vi "Hlavny program FINAL.vi"() -> ()   [LabVIEW 2018]
uses:
  <vilib>/Utility/file.llb/Write Delimited Spreadsheet (DBL).vi
panel:
  out "Pomer":dbl
  out "ERR Inicial":bool
  out "ERR VISA FUN GEN":bool
  out "ERR VISA DAQ":bool
  out "Err konveryia na string":bool
  out "size(s)":i32
  out "(HB)max":dbl
  out "Retentivita":dbl
  out "Koercitivne pole":dbl
  out "Magneticka indukcia":dbl[](array[numeric])
  out "indukovane napatie":dbl[](array[numeric])
  out "Intezita mag pola":dbl[](array[numeric])
  out "Budiac prud":dbl[](array[numeric])
  in  "File IO":bool
  out "String fun gen idn?":string
  in  "FUN GEN IDN?":bool
  in  "VISA FUN GEN":refnum<visa-resource-name>
  out "Pocet bodov":dbl
  out "Data user defined":string
  in  "Vlastny priebeh":bool
  in  "Typ priebehu":string(combo)="0"
  in  "Frekvencia":i16(knob)=500 scale=0.0..600.0
  in  "Magnetovací prúd":dbl(knob)=0.5 scale=0.0..1.5 scale format="%#_2f"
  out "Pocet ERR":dbl
  out "Intenzita mag. pola":waveform(dbl)(graph)
  out "ERR 2":bool
  out "DATA":string
  out "ERR 1":bool
  in  "N2":dbl=20.0
  in  "N1":dbl=131.0
  in  "h":dbl=0.005
  in  "r2":dbl=0.0125
  in  "r1":dbl=0.01
  in  "Rn":dbl=4.7
  in  "Demangnetizacia":bool
  out "Slucka":cluster{dbl, dbl}[](graph)
  out "String":string
  in  "daq IDN?":bool
  out "Indukuvane napatie":waveform(dbl)(graph)
  out "Magneticka indukcia":waveform(dbl)(graph)
  out "Budiaci prud":waveform(dbl)(graph)
  in  "DAQ":refnum<visa-resource-name>
  in  "Meranie":bool
  in  "stop":bool
  # "Prametre vzorky"
  # "Uh*N1"
  # "2*Pi"
  # "2*pi*rs"
  # "2*pi*rs*Rn"
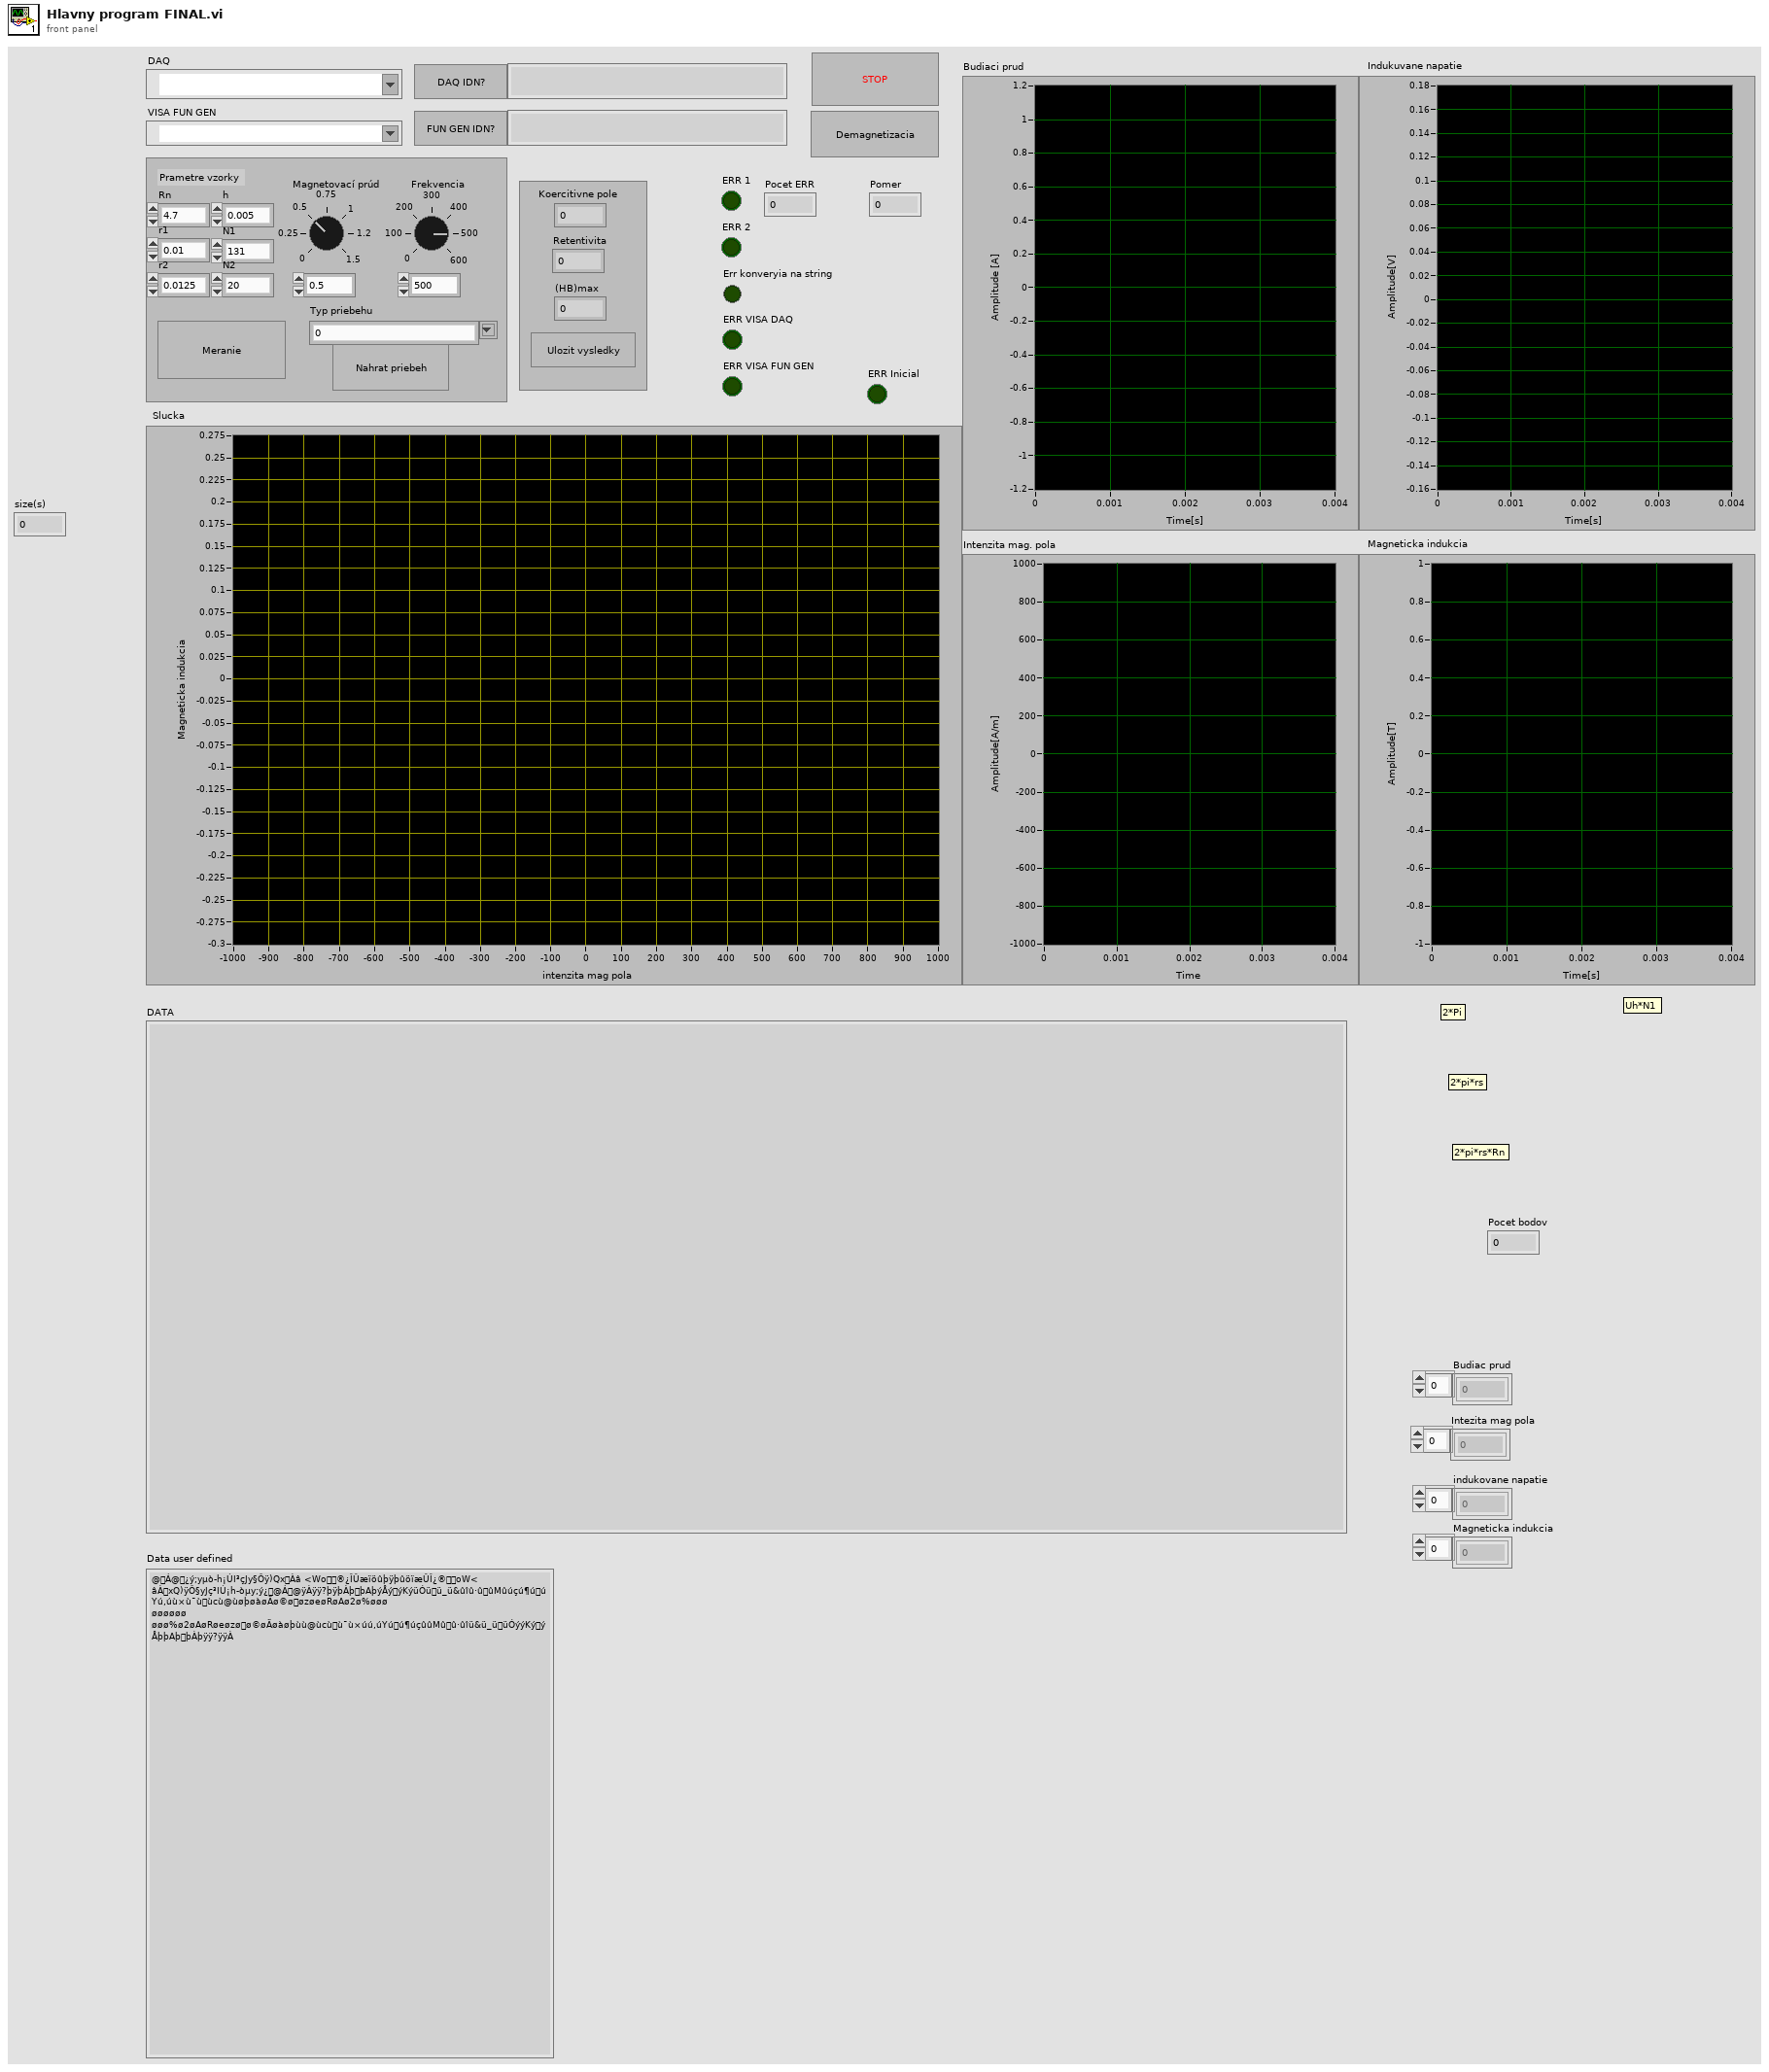
[diagram p1: front panel]
types:
  T1 = enum16{"big-endian, network order", "native, host order", "little-endian"}
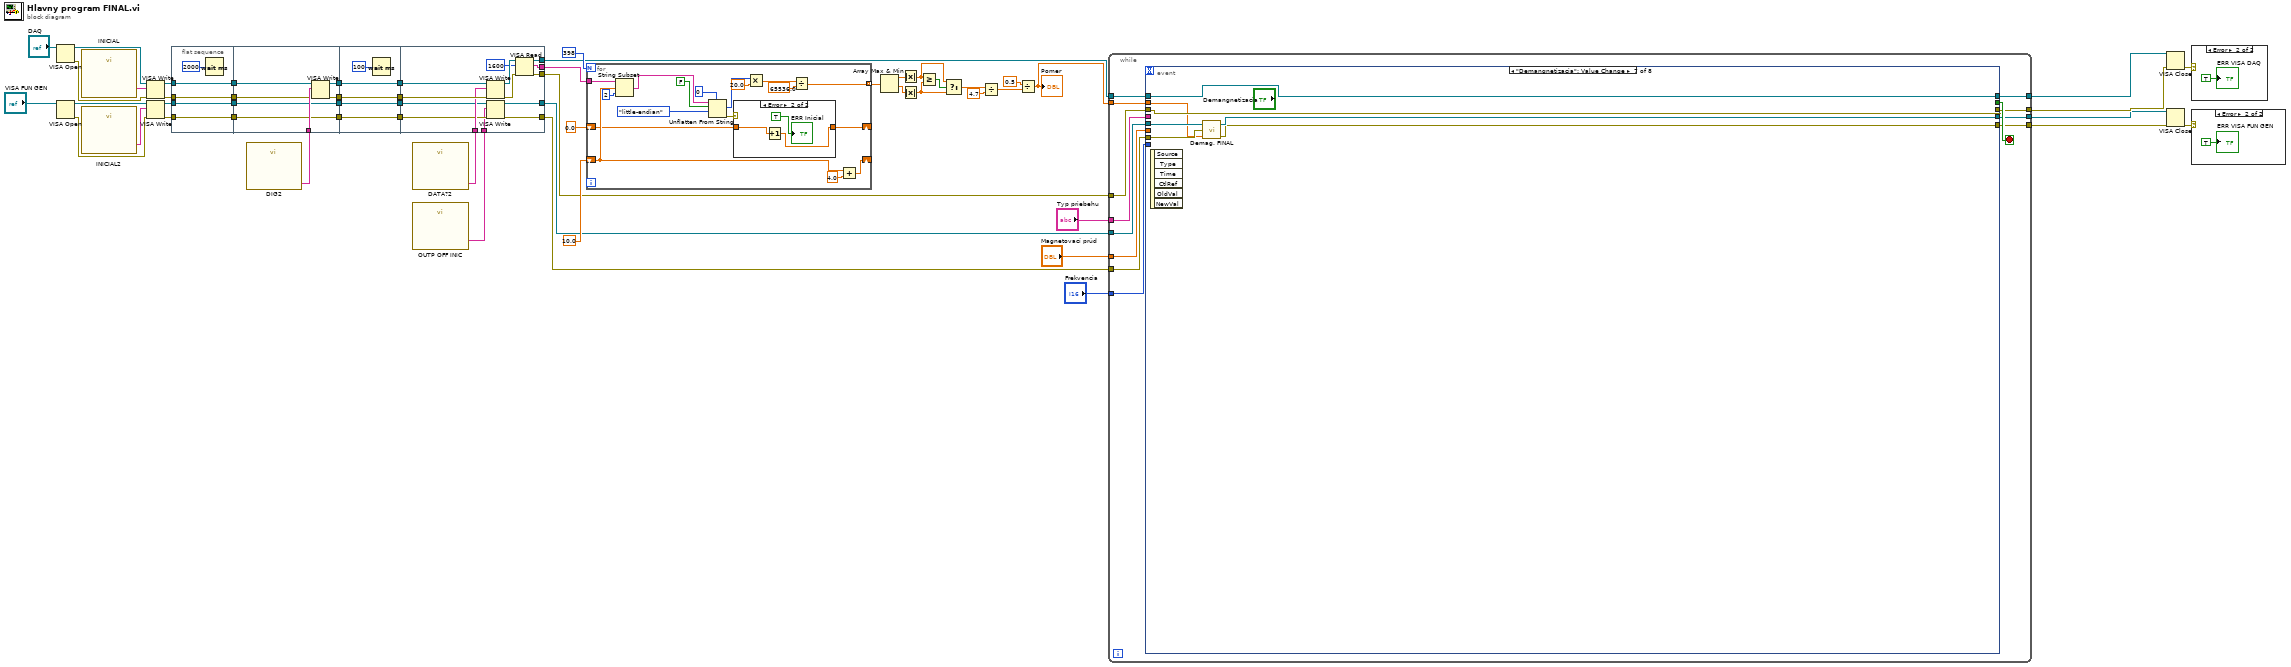
[diagram p0: block diagram]
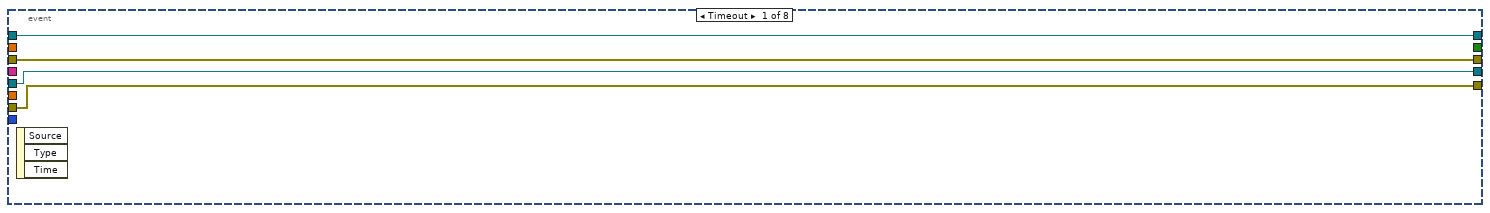
[diagram p5: hidden frame]
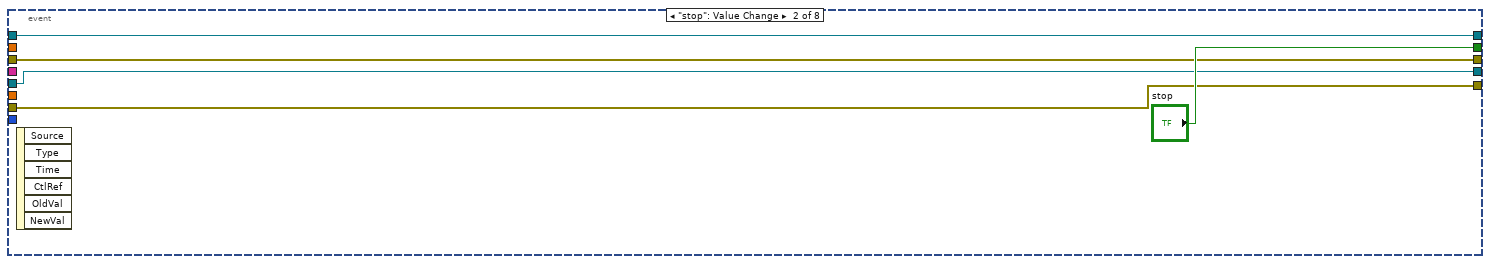
[diagram p6: hidden frame]
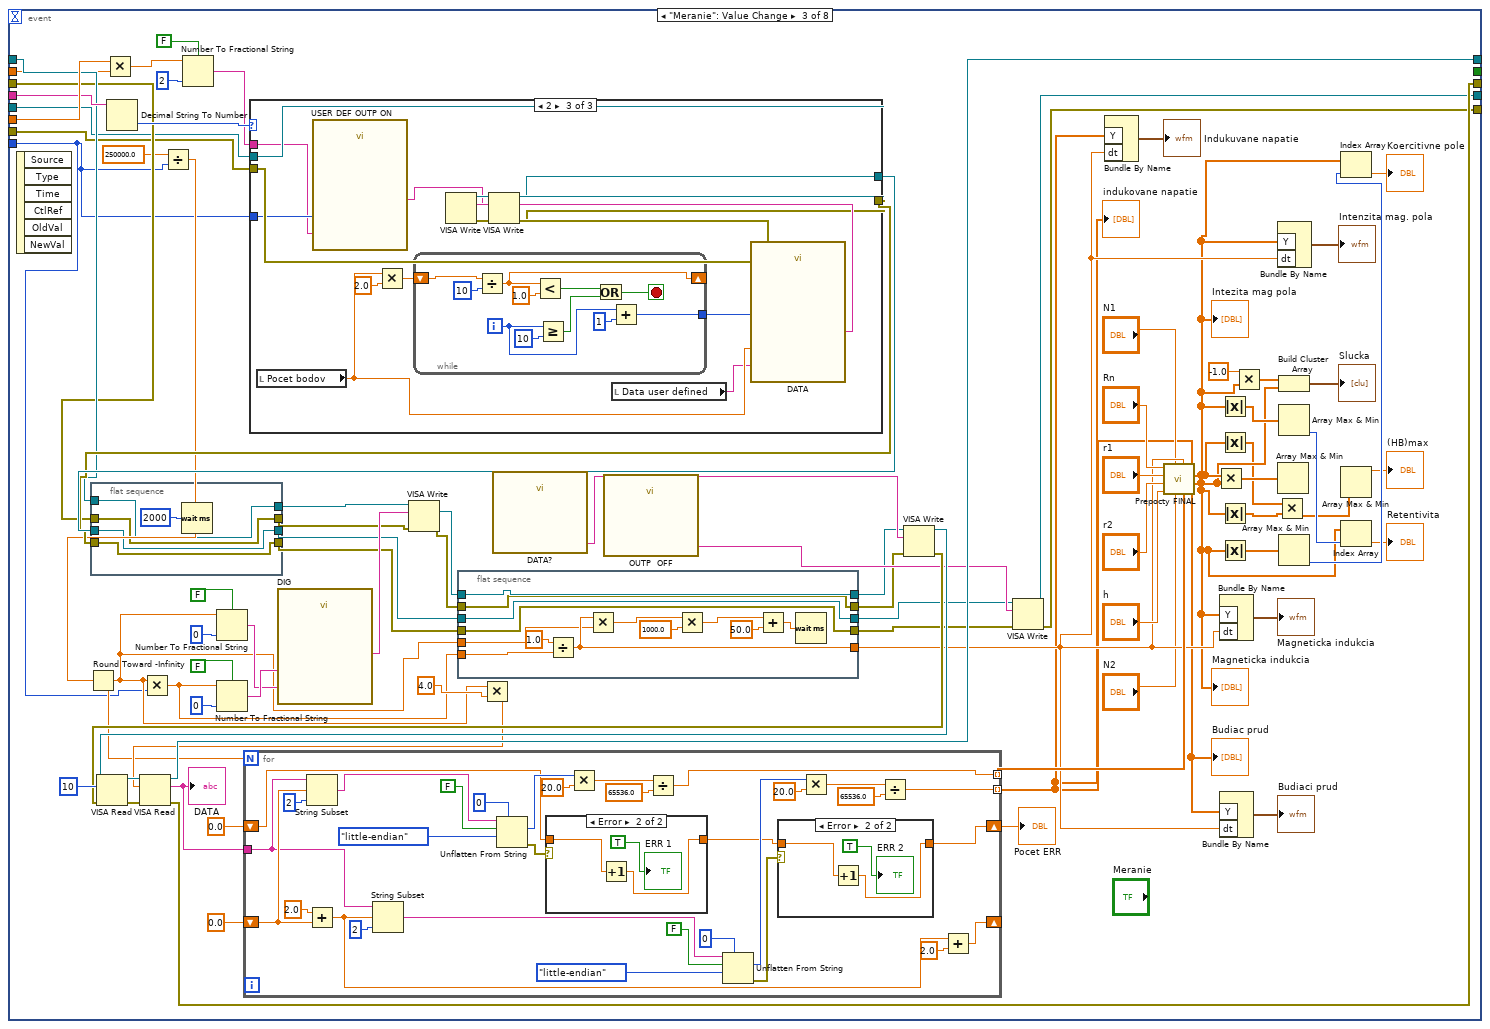
[diagram p7: hidden frame]
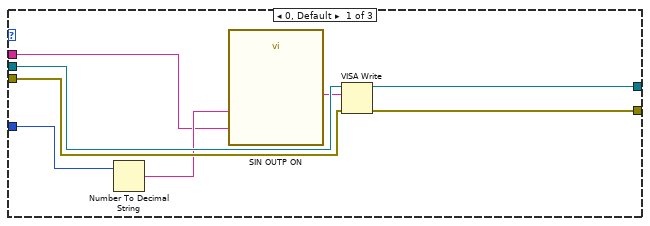
[diagram p8: hidden frame]
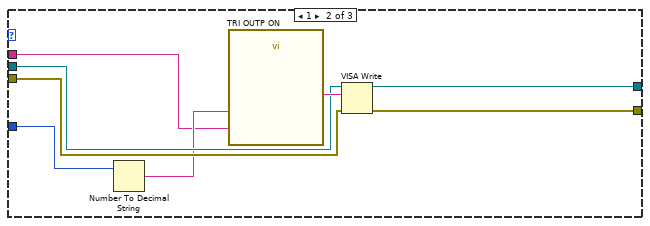
[diagram p9: hidden frame]
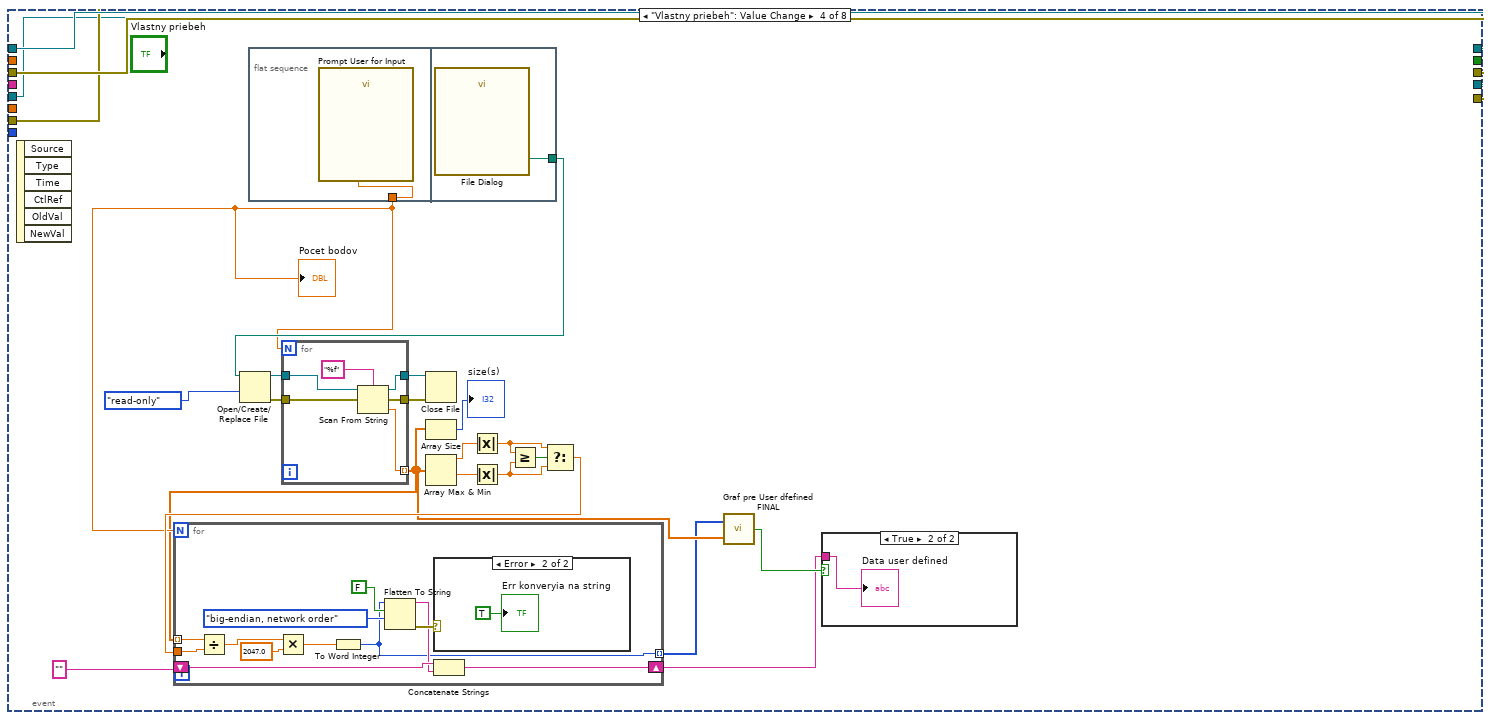
[diagram p12: hidden frame]
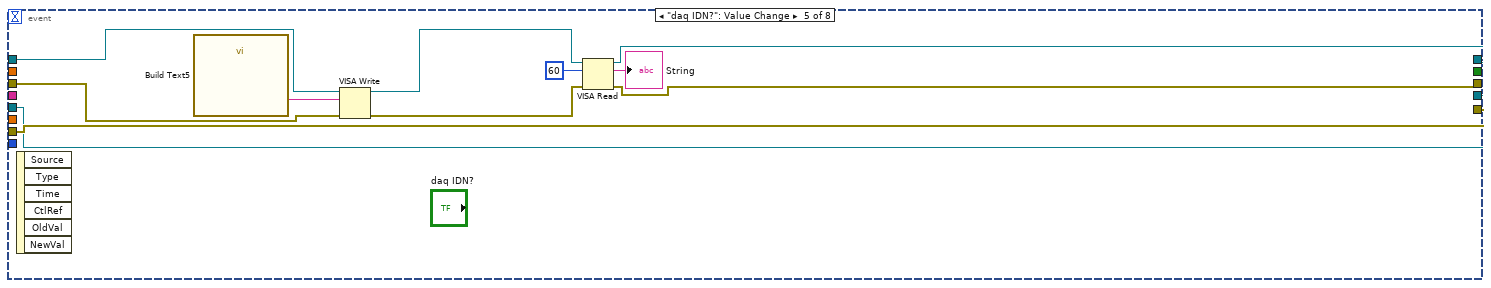
[diagram p15: hidden frame]
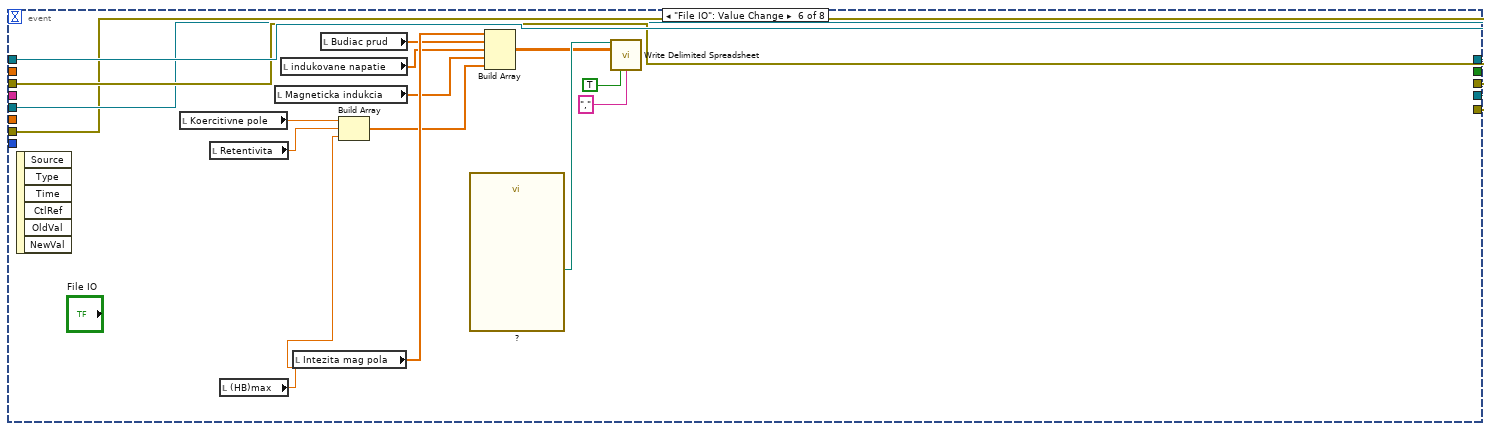
[diagram p16: hidden frame]
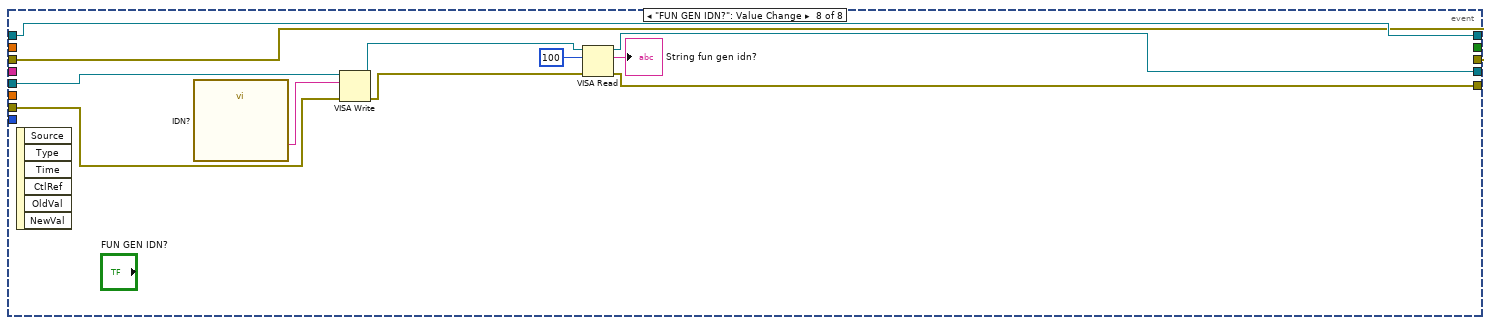
[diagram p17: hidden frame]
diagram:
  n1 = VISA Open(VISA resource name="DAQ") -> (VISA resource name=w52:refnum<visa-resource-name>, error out=w51:errorcluster)  [unwired: 4 in]
  n2 = VISA Open(VISA resource name="VISA FUN GEN") -> (VISA resource name=w43:refnum<visa-resource-name>, error out=w42:errorcluster)  [unwired: 4 in]
  n3 = call "INICIAL"() -> ("Result"=w50:string)  [unwired: 14 in, 1 out]
  n4 = call "INICIAL2"() -> ("Result"=w41:string)  [unwired: 14 in, 1 out]
  n5 = VISA Write(VISA resource name=w52, write buffer=w50, error in (no error)=w51) -> (VISA resource name out=w12:refnum<visa-resource-name>, error out=w13:errorcluster)  [unwired: 1 out]
  n6 = VISA Write(VISA resource name=w43, write buffer=w41, error in (no error)=w42) -> (VISA resource name out=w11:refnum<visa-resource-name>, error out=w10:errorcluster)  [unwired: 1 out]
  n7 = flat-sequence {
    tunnel: [w59] -> w38
    tunnel: w13 -> [w59]
    tunnel: [w58] -> w37
    tunnel: w12 -> [w58]
    tunnel: [w57] -> w36
    tunnel: w11 -> [w57]
    tunnel: [w56] -> w35
    tunnel: w10 -> [w56]
    tunnel: w26 -> [w67]
    tunnel: w38 -> [w66]
    tunnel: w37 -> [w64]
    tunnel: [w65] -> w34
    tunnel: [w63] -> w33
    tunnel: [w62] -> w32
    tunnel: w36 -> [w62]
    tunnel: [w61] -> w31
    tunnel: w35 -> [w61]
    tunnel: w34 -> [w72]
    tunnel: w33 -> [w71]
    tunnel: [w72] -> w30
    tunnel: [w71] -> w29
    tunnel: [w69] -> w28
    tunnel: w32 -> [w69]
    tunnel: [w68] -> w27
    tunnel: w31 -> [w68]
    tunnel: w30 -> [w85]
    tunnel: w29 -> [w86]
    tunnel: w25 -> [w84]
    tunnel: [w80] -> w24
    tunnel: [w79] -> w5
    tunnel: [w78] -> w6
    tunnel: w28 -> [w77]
    tunnel: w27 -> [w76]
    tunnel: [w75] -> w3
    tunnel: [w74] -> w4
    tunnel: w21 -> [w73]
    frame #0 {
      n8 = Wait (ms)(milliseconds to wait=u32 2000) -> ()  [unwired: 1 out]
    }
    frame #1 {
      n9 = VISA Write(VISA resource name=w64, write buffer=w67, error in (no error)=w66) -> (VISA resource name out=w63:refnum<visa-resource-name>, error out=w65:errorcluster)  [unwired: 1 out]
    }
    frame #2 {
      n10 = Wait (ms)(milliseconds to wait=u32 100) -> ()  [unwired: 1 out]
    }
    frame #3 {
      n11 = VISA Write(VISA resource name=w86, write buffer=w84, error in (no error)=w85) -> (VISA resource name out=w83:refnum<visa-resource-name>, error out=w82:errorcluster)  [unwired: 1 out]
      n12 = VISA Write(VISA resource name=w77, write buffer=w73, error in (no error)=w76) -> (VISA resource name out=w75:refnum<visa-resource-name>, error out=w74:errorcluster)  [unwired: 1 out]
      n13 = VISA Read(VISA resource name=w83, byte count=u32 1600, error in (no error)=w82) -> (VISA resource name out=w79:refnum<visa-resource-name>, read buffer=w80:string, error out=w78:errorcluster)  [unwired: 1 out]
    }
  }
  n14 = call "DIG2"() -> ("Result"=w26:string)  [unwired: 14 in, 1 out]
  n15 = call "DATA?2"() -> ("Result"=w25:string)  [unwired: 14 in, 1 out]
  n16 = call "OUTP OFF INIC"() -> ("Result"=w21:string)  [unwired: 14 in, 1 out]
  n17 = for {
    N: 398 -> [_]
    shift-right: [w102] -> _
    shift-left: 10.0 -> [w88]
    shift-right: [w92] -> _
    shift-left: 0.0 -> [w87]
    tunnel: w24 -> [w89]
    tunnel: [w90] -> w2 mode=indexing
    n18 = String Subset(string=w89, offset (0)=w88, length (rest)=2 ("length (rest)")) -> (substring=w93:string)
    n19 = Unflatten From String(type=i16 0, binary string=w93, data includes array or string size? (T)=FALSE, byte order (0:big-endian, network order)=T1."little-endian") -> (value=w96:i16, error out=w91:errorcluster)  [unwired: 1 in, 1 out]
    n20 = case shown="Error" w91 {
      tunnel: [w104 w106] -> w92
      tunnel: w87 -> [w104 w105]
      frame No Error {
      }
      frame Error {
        n21 = Increment(x=w105) -> (x+1=w106:dbl)
        "ERR Inicial" <- TRUE ("ERR")
      }
    }
    n22 = Multiply(x=w96, y=20.0) -> (x*y=w100:dbl)
    n23 = Divide(x=w100, y=65536.0) -> (x/y=w90:dbl)
    n24 = Add(x=w88, y=4.0) -> (x+y=w102:dbl)
  }
  n25 = Array Max & Min(array=w2) -> (max value=w20:dbl, min value=w19:dbl)  [unwired: 2 out]
  n26 = Absolute Value(x=w20) -> (abs(x)=w18:dbl)
  n27 = Absolute Value(x=w19) -> (abs(x)=w17:dbl)
  n28 = Greater Or Equal?(x=w18, y=w17) -> (x >= y?=w16:bool)
  n29 = Select(t=w18, s=w16, f=w17) -> (s? t:f=w9:dbl)
  n30 = Divide(x=w9, y=4.7) -> (x/y=w7:dbl)
  n31 = Divide(x=0.5, y=w7) -> (x/y=w1:dbl)
  "Pomer" <- w1
  n32 = while {
    tunnel: w5 -> [w119]
    tunnel: w6 -> [w118]
    tunnel: [w117] -> w54
    tunnel: [w116] -> w53
    tunnel: "Magnetovací prúd" -> [w115]
    tunnel: "Frekvencia" -> [w113]
    tunnel: "Typ priebehu" -> [w114]
    tunnel: w3 -> [w112]
    tunnel: w4 -> [w111]
    tunnel: [w110] -> w45
    tunnel: [w109] -> w44
    tunnel: w1 -> [w108]
    stop <- w120 stop-if-true
    n33 = event shown="[6] \"Demangnetizacia\": Value Change" {
      selector: _ -> [_ _ _ _ _ _ _ _]
      dyn-events: _ -> [_ _ _ _ _ _ _ _]
      timeout: _ -> [_ _ _ _ _ _ _ _]
      tunnel: [_ "stop" _ _ _ _ _ _] -> w120
      tunnel: w119 -> [w124 w128 w170 w333 w367 w383 w390 w401]
      tunnel: w118 -> [w121 w125 w168 w334 w366 w382 w389 w397]
      tunnel: [w124 w128 w198 w333 w360 w383 w390 w401] -> w117
      tunnel: [w121 w125 w197 w334 w359 w382 w389 w397] -> w116
      tunnel: w115 -> [_ _ w187 _ _ _ _ _]
      tunnel: w114 -> [_ _ w186 _ _ _ _ _]
      tunnel: w113 -> [_ _ w131 _ _ _ _ _]
      tunnel: w112 -> [w122 w126 w165 w330 w357 w381 w388 w399]
      tunnel: w111 -> [w123 w127 w164 w331 w358 w380 w387 w398]
      tunnel: [w122 w126 w158 w330 w357 w381 w386 w394] -> w110
      tunnel: [w123 w127 w159 w331 w358 w380 w385 w393] -> w109
      tunnel: w108 -> [_ _ w130 _ _ _ w384 _]
      event Timeout {
        n34 = event-data() -> ()  [unwired: 1 in, 3 out]
      }
      event "stop": Value Change {
        n35 = event-data() -> ()  [unwired: 1 in, 6 out]
      }
      event "Meranie": Value Change {
        n36 = event-data() -> ()  [unwired: 1 in, 6 out]
        n37 = flat-sequence {
          tunnel: [w311] -> w161
          tunnel: w183 -> [w311]
          tunnel: [w310] -> w162
          tunnel: w182 -> [w310]
          tunnel: [w308] -> w171
          tunnel: w170 -> [w308]
          tunnel: [w307] -> w169
          tunnel: w168 -> [w307]
          frame #0 {
            n38 = Wait (ms)(milliseconds to wait=u32 2000) -> ()  [unwired: 1 out]
          }
        }
        n39 = Multiply(x=w187, y=w130) -> (x*y=w188:dbl)
        n40 = Decimal String To Number(string=w186) -> (number=w185:i32)  [unwired: 2 in, 1 out]
        n41 = Divide(x=250000.0, y=w131) -> (x/y=w142:dbl)
        n42 = Round Toward -Infinity(1:w142) -> (0:w133:dbl)
        n43 = Multiply(x=w133, y=w131) -> (x*y=w132:dbl)
        n44 = Number To Fractional String(use system decimal point (T)=FALSE, number=w188, precision (6)=i16 2) -> (F-format string=w184:string)  [unwired: 1 in]
        n45 = Number To Fractional String(use system decimal point (T)=FALSE, number=w133, precision (6)=i16 0) -> (F-format string=w137:string)  [unwired: 1 in]
        n46 = Number To Fractional String(use system decimal point (T)=FALSE, number=w132, precision (6)=i16 0) -> (F-format string=w138:string)  [unwired: 1 in]
        n47 = case shown="2" w185 {
          tunnel: w184 -> [w213 w221 w229]
          tunnel: w164 -> [w219 w226 w242]
          tunnel: w165 -> [w218 w225 w243]
          tunnel: [w216 w223 w238] -> w183
          tunnel: [w217 w224 w237] -> w182
          tunnel: w131 -> [w220 w228 w230]
          frame 0, Default {
            n48 = Number To Decimal String(number=w220) -> (decimal integer string=w214:string)  [unwired: 1 in]
            n49 = call "SIN OUTP ON"("Frekv"=w214, "ampl"=w213) -> ("Result"=w215:string)  [unwired: 12 in, 1 out]
            n50 = VISA Write(VISA resource name=w218, write buffer=w215, error in (no error)=w219) -> (VISA resource name out=w216:refnum<visa-resource-name>, error out=w217:errorcluster)  [unwired: 1 out]
          }
          frame 1 {
            n51 = Number To Decimal String(number=w228) -> (decimal integer string=w222:string)  [unwired: 1 in]
            n52 = call "TRI OUTP ON"("Frekv"=w222, "ampl"=w221) -> ("Result"=w227:string)  [unwired: 12 in, 1 out]
            n53 = VISA Write(VISA resource name=w225, write buffer=w227, error in (no error)=w226) -> (VISA resource name out=w223:refnum<visa-resource-name>, error out=w224:errorcluster)  [unwired: 1 out]
          }
          frame 2 {
            n54 = local read "Pocet bodov"() -> (w233:dbl)
            n55 = call "USER DEF OUTP ON"("frekv"=w230, "ampl"=w229) -> ("Result"=w236:string)  [unwired: 12 in, 1 out]
            n56 = Multiply(x=w233, y=2.0) -> (x*y=w234:dbl)
            n57 = while {
              shift-right: [w247] -> _
              shift-left: w234 -> [w249]
              tunnel: [w244] -> w231
              i -> [w246]
              stop <- w250 stop-if-true
              n58 = Divide(x=w249, y=10) -> (x/y=w247:dbl)
              n59 = Less?(x=w247, y=1.0) -> (x < y?=w253:bool)
              n60 = Greater Or Equal?(x=w246, y=10) -> (x >= y?=w252:bool)
              n61 = Or(x=w253, y=w252) -> (x .or. y?=w250:bool)
              n62 = Add(x=w246, y=1) -> (x+y=w244:i32)
            }
            n63 = local read "Data user defined"() -> (w232:string)
            n64 = call "DATA"("pocetdig"=w231, "pocetbod"=w233, "data"=w232) -> ("Result"=w241:string)  [unwired: 11 in, 1 out]
            n65 = VISA Write(VISA resource name=w243, write buffer=w241, error in (no error)=w242) -> (VISA resource name out=w240:refnum<visa-resource-name>, error out=w239:errorcluster)  [unwired: 1 out]
            n66 = VISA Write(VISA resource name=w240, write buffer=w236, error in (no error)=w239) -> (VISA resource name out=w238:refnum<visa-resource-name>, error out=w237:errorcluster)  [unwired: 1 out]
          }
        }
        n67 = call "DIG"("frekv"=w138, "body"=w137) -> ("Result"=w212:string)  [unwired: 12 in, 1 out]
        n68 = VISA Write(VISA resource name=w171, write buffer=w212, error in (no error)=w169) -> (VISA resource name out=w211:refnum<visa-resource-name>, error out=w210:errorcluster)  [unwired: 1 out]
        n69 = flat-sequence {
          tunnel: w211 -> [w303]
          tunnel: [w303] -> w167
          tunnel: w210 -> [w302]
          tunnel: [w302] -> w166
          tunnel: [w301] -> w176
          tunnel: [w297] -> w163
          tunnel: w162 -> [w297]
          tunnel: [w296] -> w160
          tunnel: w161 -> [w296]
          tunnel: w132 -> [w295]
          tunnel: w133 -> [w294]
          frame #0 {
            n70 = Divide(x=1.0, y=w295) -> (x/y=w301:dbl)
            n71 = Multiply(x=w301, y=w294) -> (x*y=w300:dbl)
            n72 = Multiply(x=w300, y=1000.0) -> (x*y=w298:dbl)
            n73 = Add(x=w298, y=50.0) -> (x+y=w304:dbl)
            n74 = Wait (ms)(milliseconds to wait=w304) -> ()  [unwired: 1 out]
          }
        }
        n75 = Multiply(x=w133, y=4.0) -> (x*y=w134:dbl)
        n76 = call "DATA?"() -> ("Result"=w196:string)  [unwired: 14 in, 1 out]
        n77 = call "OUTP  OFF"() -> ("Result"=w195:string)  [unwired: 14 in, 1 out]
        n78 = VISA Write(VISA resource name=w167, write buffer=w196, error in (no error)=w166) -> (VISA resource name out=w204:refnum<visa-resource-name>, error out=w203:errorcluster)  [unwired: 1 out]
        n79 = VISA Read(VISA resource name=w204, byte count=u32 10, error in (no error)=w203) -> (VISA resource name out=w202:refnum<visa-resource-name>, error out=w201:errorcluster)  [unwired: 2 out]
        n80 = VISA Read(VISA resource name=w202, byte count=w134, error in (no error)=w201) -> (VISA resource name out=w198:refnum<visa-resource-name>, read buffer=w194:string, error out=w197:errorcluster)  [unwired: 1 out]
        "DATA" <- w194
        n81 = for {
          N: w133 -> [_]
          shift-right: [w277] -> _
          shift-left: 0.0 -> [w267]
          shift-right: [w261] -> w191
          shift-left: 0.0 -> [w275]
          tunnel: w194 -> [w256]
          tunnel: [w259] -> w157 mode=indexing
          tunnel: [w258] -> w177 mode=indexing
          n82 = String Subset(string=w256, offset (0)=w267, length (rest)=2 ("length (rest)")) -> (substring=w276:string)
          n83 = Add(x=2.0, y=w267) -> (x+y=w257:dbl)
          n84 = String Subset(string=w256, offset (0)=w257, length (rest)=2 ("length (rest)")) -> (substring=w264:string)
          n85 = Unflatten From String(type=i16 0, binary string=w276, data includes array or string size? (T)=FALSE, byte order (0:big-endian, network order)=T1."little-endian") -> (value=w280:i16, error out=w263:errorcluster)  [unwired: 1 in, 1 out]
          n86 = case shown="Error" w263 {
            tunnel: [w290 w292] -> w262
            tunnel: w275 -> [w290 w291]
            frame No Error {
            }
            frame Error {
              n87 = Increment(x=w291) -> (x+1=w292:dbl)
              "ERR 1" <- TRUE ("ERR")
            }
          }
          n88 = Multiply(x=w280, y=20.0) -> (x*y=w284:dbl)
          n89 = Divide(x=w284, y=65536.0) -> (x/y=w258:dbl)
          n90 = Unflatten From String(type=i16 0, binary string=w264, data includes array or string size? (T)=FALSE, byte order (0:big-endian, network order)=T1."little-endian") -> (value=w269:i16, error out=w260:errorcluster)  [unwired: 1 in, 1 out]
          n91 = case shown="Error" w260 {
            tunnel: [w286 w288] -> w261
            tunnel: w262 -> [w286 w287]
            frame No Error {
            }
            frame Error {
              n92 = Increment(x=w287) -> (x+1=w288:dbl)
              "ERR 2" <- TRUE ("ERR")
            }
          }
          n93 = Multiply(x=w269, y=20.0) -> (x*y=w273:dbl)
          n94 = Divide(x=w273, y=65536.0) -> (x/y=w259:dbl)
          n95 = Add(x=w257, y=2.0) -> (x+y=w277:dbl)
        }
        "Pocet ERR" <- w191
        "indukovane napatie" <- w157
        n96 = VISA Write(VISA resource name=w160, write buffer=w195, error in (no error)=w163) -> (VISA resource name out=w158:refnum<visa-resource-name>, error out=w159:errorcluster)  [unwired: 1 out]
        n97 = Bundle By Name("Y"=w157, "dt"=w176) -> (→"Indukuvane napatie":waveform(dbl))  [unwired: 1 in]
        n98 = call "Prepocty FINAL.vi"("Ui"=w157, "Uh"=w177, "dt"=w176, "N2"="N2", "N1"="N1", "h"="h", "r2"="r2", "r1"="r1", "Rn"="Rn") -> ("I"=w173:dbl[], "B"=w148:dbl[], "H"=w149:dbl[])
        "Budiac prud" <- w173
        "Intezita mag pola" <- w149
        "Magneticka indukcia" <- w148
        n99 = Multiply(x=w149, y=w148) -> (x*y=w150:dbl[])
        n100 = Absolute Value(x=w149) -> (abs(x)=w154:dbl[])
        n101 = Absolute Value(x=w149) -> (abs(x)=w147:dbl[])
        n102 = Absolute Value(x=w148) -> (abs(x)=w146:dbl[])
        n103 = Absolute Value(x=w148) -> (abs(x)=w156:dbl[])
        n104 = Bundle By Name("Y"=w148, "dt"=w176) -> (→"Magneticka indukcia":waveform(dbl))  [unwired: 1 in]
        n105 = Bundle By Name("Y"=w173, "dt"=w176) -> (→"Budiaci prud":waveform(dbl))  [unwired: 1 in]
        n106 = Multiply(x=-1.0, y=w149) -> (x*y=w172:dbl[])
        n107 = Multiply(x=w147, y=w146) -> (x*y=w145:dbl[])
        n108 = Bundle By Name("Y"=w149, "dt"=w176) -> (→"Intenzita mag. pola":waveform(dbl))  [unwired: 1 in]
        n109 = Array Max & Min(array=w150) -> ()  [unwired: 4 out]
        n110 = Build Cluster Array(w172, w148) -> (→"Slucka":cluster{dbl, dbl}[])
        n111 = Array Max & Min(array=w154) -> (min index (indices)=w153:i32)  [unwired: 3 out]
        n112 = Array Max & Min(array=w156) -> (min index (indices)=w155:i32)  [unwired: 3 out]
        n113 = Index Array(array=w149, index=w155) -> (element=→"Koercitivne pole":dbl)
        n114 = Array Max & Min(array=w145) -> (max value=→"(HB)max":dbl)  [unwired: 3 out]
        n115 = Index Array(array=w148, index=w153) -> (element=→"Retentivita":dbl)
      }
      event "Vlastny priebeh": Value Change {
        n116 = event-data() -> ()  [unwired: 1 in, 6 out]
        n117 = Open/Create/Replace File(file path (use dialog)=w316, access (0:read/write)=enum16{"read/write", "read-only", "write-only"}."read-only") -> (refnum out=w328:refnum<file>, error out=w327:errorcluster)  [unwired: 4 in, 1 out]
        n118 = flat-sequence {
          tunnel: [w355] -> w315
          tunnel: [w356] -> w316
          frame #0 {
            n119 = call "Prompt User for Input"() -> ("Pocet bodov"=w355:dbl)  [unwired: 17 in, 2 out]
          }
          frame #1 {
            n120 = call "File Dialog"() -> ("selected path"=w356:path)  [unwired: 12 in, 3 out]
          }
        }
        n121 = for {
          N: w315 -> [_]
          tunnel: w328 -> [w350]
          tunnel: w327 -> [w349]
          tunnel: [w353] -> w325
          tunnel: [w352] -> w326
          tunnel: [w348] -> w314 mode=indexing
          n122 = Scan From String("%f" ("format string"), w350, w349) -> (w353:refnum<file>, w352:errorcluster, output 1=w348:dbl)  [unwired: 1 in]
        }
        n123 = Close File(refnum=w325, error in=w326) -> ()  [unwired: 2 out]
        n124 = Array Size(array=w314) -> (size(s)=→"size(s)":i32)
        n125 = Array Max & Min(array=w314) -> (max value=w323:dbl, min value=w322:dbl)  [unwired: 2 out]
        n126 = Absolute Value(x=w323) -> (abs(x)=w320:dbl)
        n127 = Absolute Value(x=w322) -> (abs(x)=w319:dbl)
        n128 = Greater Or Equal?(x=w320, y=w319) -> (x >= y?=w321:bool)
        n129 = Select(t=w320, s=w321, f=w319) -> (s? t:f=w318:dbl)
        n130 = for {
          N: w315 -> [_]
          tunnel: w318 -> [w342]
          tunnel: w314 -> [w343] mode=indexing
          shift-right: [w338] -> w312
          shift-left: "" -> [w337]
          tunnel: [w335] -> w313 mode=indexing
          n131 = Divide(x=w343, y=w342) -> (x/y=w341:dbl)
          n132 = Multiply(x=w341, y=2047.0) -> (x*y=w339:dbl)
          n133 = To Word Integer(number=w339) -> (16bit integer=w335:i16)
          n134 = Flatten To String(anything=w335, prepend array or string size? (T)=FALSE, byte order (0:big-endian, network order)=T1."big-endian, network order") -> (data string=w336:string, error out=w346:errorcluster)  [unwired: 1 in, 1 out]
          n135 = case shown="Error" w346 {
            frame No Error {
            }
            frame Error {
              "Err konveryia na string" <- TRUE ("Err konveryia na string")
            }
          }
          n136 = Concatenate Strings(w337, w336) -> (w338:string)
        }
        n137 = call "Graf pre User dfefined FINAL.vi"("Array"=w314, "Array 2"=w313) -> ("Boolean"=w332:bool)
        n138 = case shown="True" w332 {
          tunnel: w312 -> [_ w354]
          frame False {
          }
          frame True {
            "Data user defined" <- w354
          }
        }
        "Pocet bodov" <- w315
      }
      event "daq IDN?": Value Change {
        n139 = event-data() -> ()  [unwired: 1 in, 6 out]
        n140 = call "Build Text5"() -> ("Result"=w363:string)  [unwired: 14 in, 1 out]
        n141 = VISA Write(VISA resource name=w367, write buffer=w363, error in (no error)=w366) -> (VISA resource name out=w365:refnum<visa-resource-name>, error out=w364:errorcluster)  [unwired: 1 out]
        n142 = VISA Read(VISA resource name=w365, byte count=u32 60, error in (no error)=w364) -> (VISA resource name out=w360:refnum<visa-resource-name>, read buffer=→"String":string, error out=w359:errorcluster)  [unwired: 1 out]
      }
      event "File IO": Value Change {
        n143 = event-data() -> ()  [unwired: 1 in, 6 out]
        n144 = local read "Koercitivne pole"() -> (w371:dbl)
        n145 = local read "Retentivita"() -> (w370:dbl)
        n146 = local read "(HB)max"() -> (w369:dbl)
        n147 = local read "Magneticka indukcia"() -> (w373:dbl[])
        n148 = local read "indukovane napatie"() -> (w374:dbl[])
        n149 = local read "Intezita mag pola"() -> (w376:dbl[])
        n150 = local read "Budiac prud"() -> (w375:dbl[])
        n151 = Build Array(w371, w370, w369) -> (w368:dbl[])
        n152 = call "?"() -> ("selected path"=w379:path)  [unwired: 12 in, 3 out]
        n153 = Build Array(w376, w375, w374, w373, w368) -> (w372:dbl[][])
        n154 = call-poly <vilib>:"Write Delimited Spreadsheet.vi"("file path (dialog if empty)"=w379, "2D data"=w372, "transpose? (no:F)"=TRUE, "delimiter (\\t)"="," ("delimiter (\\t)")) -> ()  [unwired: 10 in, 2 out]
      }
      event "Demangnetizacia": Value Change {
        n155 = event-data() -> ()  [unwired: 1 in, 6 out]
        n156 = call "Demag. FINAL.vi"("pomer"=w384, "error in (no error) FUN GEN"=w387, "VISA resource name FUN GEN"=w388) -> ("error out FUN GEN"=w385:errorcluster, "VISA resource name out FUN GEN"=w386:refnum<visa-resource-name>)  [unwired: 1 out]
      }
      event "FUN GEN IDN?": Value Change {
        n157 = event-data() -> ()  [unwired: 1 in, 6 out]
        n158 = call "IDN?"() -> ("Result"=w400:string)  [unwired: 14 in, 1 out]
        n159 = VISA Write(VISA resource name=w399, write buffer=w400, error in (no error)=w398) -> (VISA resource name out=w396:refnum<visa-resource-name>, error out=w395:errorcluster)  [unwired: 1 out]
        n160 = VISA Read(VISA resource name=w396, byte count=u32 100, error in (no error)=w395) -> (VISA resource name out=w394:refnum<visa-resource-name>, read buffer=→"String fun gen idn?":string, error out=w393:errorcluster)  [unwired: 1 out]
      }
    }
  }
  n161 = VISA Close(VISA resource name=w54, error in (no error)=w53) -> (error out=w40:errorcluster)
  n162 = VISA Close(VISA resource name=w45, error in (no error)=w44) -> (error out=w39:errorcluster)
  n163 = case shown="Error" w40 {
    frame No Error {
    }
    frame Error {
      "ERR VISA DAQ" <- TRUE ("ERR VISA DAQ")
    }
  }
  n164 = case shown="Error" w39 {
    frame No Error {
    }
    frame Error {
      "ERR VISA FUN GEN" <- TRUE ("ERR VISA FUN GEN")
    }
  }
